vi "StopAcquisition.vi"(8 "error in (no error)":errorcluster, 11 "reference in":refnum<class "Camera_Sim.lvclass">) -> (0 "error out":errorcluster, 3 "reference out":refnum<class "Camera_Sim.lvclass">)   [LabVIEW 2017, in "Camera_Sim.lvclass"]
uses:
  Camera_Sim.lvclass
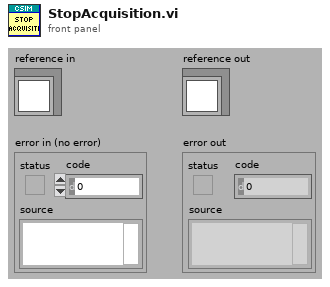
[diagram p1: front panel]
types:
  T1 = typedef "CameraSim.lvclass/ObjectAttributes.ctl" = cluster{"Connected":bool, "Image Out":T2, "Frame Number":u32, "Path":path}
  T2 = typedef "IMAQ Image.ctl" = refnum<image>
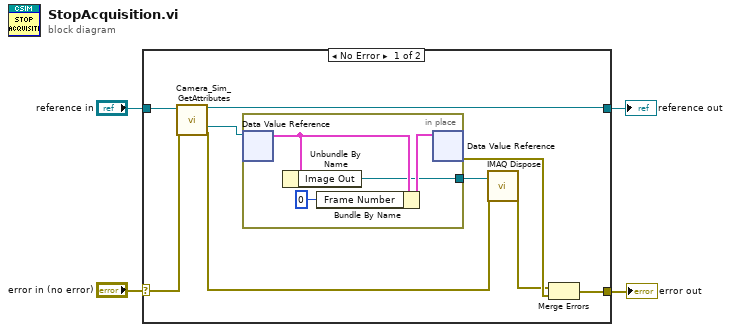
[diagram p0: block diagram]
diagram:
  n1 = case shown="No Error" "error in (no error)" {
    selector: "error in (no error)" -> [w12 w19]
    tunnel: [w9 w19] -> w3
    tunnel: [w8 w18] -> w1
    tunnel: "reference in" -> [w13 w18]
    frame No Error {
      n2 = call "Camera_Sim_GetAttributes.vi"("reference in"=w13, "error in (no error)"=w12) -> ("reference out"=w8:refnum<class "Camera_Sim.lvclass">, "DataRef"=w10:refnum<data-value>, "error out"=w6:errorcluster)  [unwired: 10 in, 1 out]
      n3 = in-place {
        in-place-border: [w14] -> w7
        n4 = in-place-dvr #1(w10) -> (w15:T1)  [unwired: 1 out]
        n5 = Unbundle By Name(w15) -> ("Image Out"=w14:T2)
        n6 = Bundle By Name(cluster=w15, "Frame Number"=u32 0) -> (w17:T1)
        n7 = in-place-dvr #1(w17) -> (w11:errorcluster)  [unwired: 1 out]
      }
      n8 = call "IMAQ Dispose"("Image"=w7, "error in (no error)"=w6) -> ("error out"=w5:errorcluster)  [unwired: 4 in]
      n9 = Merge Errors(w5, w11) -> (w9:errorcluster)
    }
    frame Error {
    }
  }
  "error out" <- w3
  "reference out" <- w1
